vi "APS arc2 ce.vi"(0 "Axis_ID_Array":i32, 1 "Option":i32, 2 "CenterArray":dbl, 3 "EndArray":dbl, 4 "Dir":i16, 5 "TransPara":dbl, 6 "Wait":cluster{"h_event":u32, "i32_ret":i32}, 7 "error in (no error)":errorcluster caption="错误输入（无错误）") -> (20 "Axis_ID_Array out":i32, 21 "function return":i32, 22 "CenterArray out":dbl, 23 "EndArray out":dbl, 25 "TransPara out":dbl, 26 "Wait out":cluster{"h_event":u32, "i32_ret":i32}, 27 "error out":errorcluster caption="错误输出")   [LabVIEW 2011, in "APS168.lvlib"]
doc: "I32 FNTYPE APS_arc2_ce( I32 *Axis_ID_Array, I32 Option, F64 *CenterArray, F64 *EndArray, I16 Dir, F64 *TransPara, ASYNCALL *Wait );"
uses:
  APS168.lvlib
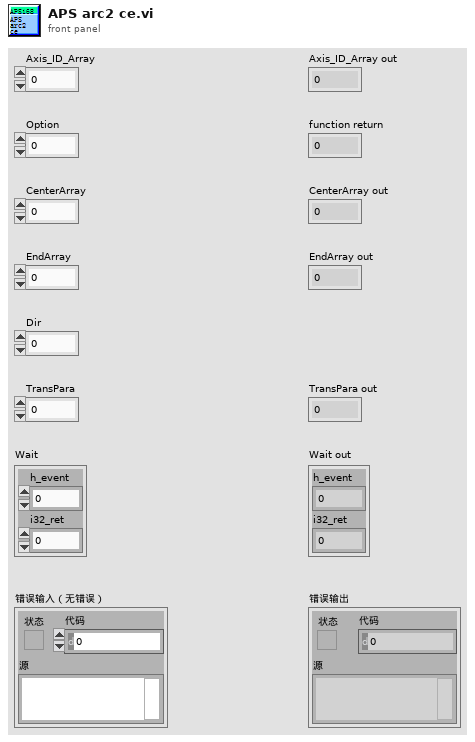
[diagram p1: front panel]
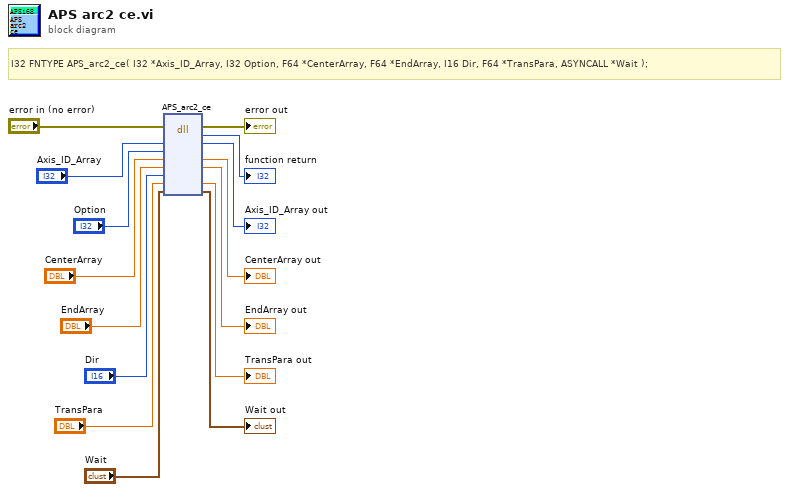
[diagram p0: block diagram]
diagram:
  # "I32 FNTYPE APS_arc2_ce( I32 *Axis_ID_Array, I32 Option, F64 *CenterArray, F64 *EndArray, I16 Dir, F64 *TransPara, ASYNCALL *Wait );"
  n1 = dll-call lib="PTH1Labs E软件ADLINK 204CAPS_1_7_1_LIB line 连续运动204APS168.*" fn="APS_arc2_ce"(error in="error in (no error)", "Axis_ID_Array"="Axis_ID_Array", "Option"="Option", "CenterArray"="CenterArray", "EndArray"="EndArray", "Dir"="Dir", "TransPara"="TransPara", "Wait"="Wait") -> (error out=→"error out":errorcluster, →"function return":i32, "Axis_ID_Array"=→"Axis_ID_Array out":i32, "CenterArray"=→"CenterArray out":dbl, "EndArray"=→"EndArray out":dbl, "TransPara"=→"TransPara out":dbl, "Wait"=→"Wait out":cluster{"h_event":u32, "i32_ret":i32})  [unwired: 4 in, 1 out]
